vi "Format 2D.vi"(1 "2D Array":dbl[][](array[numeric]), 2 "2D Array name":string) -> (0 "String":string)   [LabVIEW 2016, in "LV to ITX.lvclass"]
uses:
  LV to ITX.lvclass
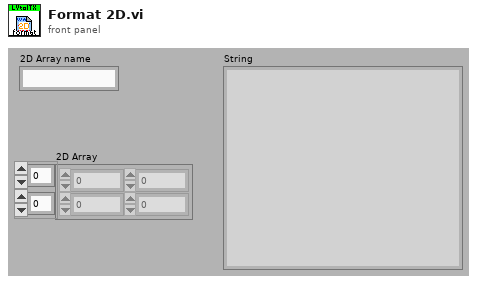
[diagram p1: front panel]
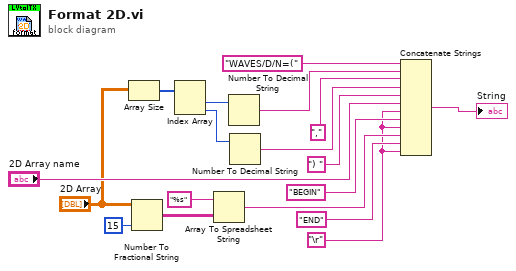
[diagram p0: block diagram]
diagram:
  w2 = "\r"
  n1 = Array Size(array="2D Array") -> (size(s)=w7:i32[])
  n2 = Number To Fractional String(number="2D Array", precision (6)=i16 15) -> (F-format string=w4:string[][])  [unwired: 2 out]
  n3 = Index Array(array=w7) -> (element #1=w8:i32, element #2=w9:i32)  [unwired: 2 in]
  n4 = Array To Spreadsheet String(array=w4, 3:"%s" ("format string")) -> (spreadsheet string=w12:string)  [unwired: 1 out]
  n5 = Number To Decimal String(number=w8) -> (decimal integer string=w17:string)  [unwired: 1 out]
  n6 = Number To Decimal String(number=w9) -> (decimal integer string=w15:string)  [unwired: 1 out]
  n7 = Concatenate Strings("WAVES/D/N=(", w17, ",", w15, ") ", "2D Array name", w2, "BEGIN", w2, w12, "END", w2) -> (→"String":string)
